vi "Transmitted Bytes.vi"(11 "Additional":i32) -> (3 "Tally":i32)   [LabVIEW 2017]
doc: "Add to the running total of bytes transmitted as part of the NT protocol."
uses:
  <vilib>/Rock Robotics/Network Tables/NT Globals.vi
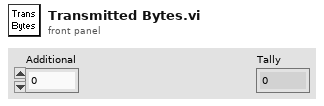
[diagram p1: front panel]
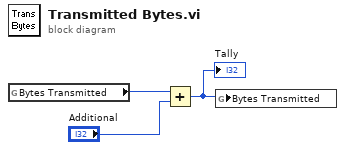
[diagram p0: block diagram]
diagram:
  n1 = global read "NT Globals.vi" "Bytes Transmitted"() -> (w3:i32)
  n2 = Add(x=w3, y="Additional") -> (x+y=w1:i32)
  "Tally" <- w1
  n3 = global write "NT Globals.vi" "Bytes Transmitted"(w1) -> ()
